vi "convolution.vi"() -> ()   [LabVIEW 2015]
uses:
  <vilib>/vision/NI_Vision_Development_Module.lvlib
panel:
  out "Kernel":dbl[][][](array[numeric])
  out "Image 5":T1(plugin-control)
  out "Image 4":T1(plugin-control)
  out "kernel2":dbl[][](array[numeric])
  out "Divider2":dbl
  out "Divider1":dbl
  out "kernel1":dbl[][](array[numeric])
  out "Image 3":T1(plugin-control)
  out "ImageSize":i32=500
  out "Image":T1(plugin-control)
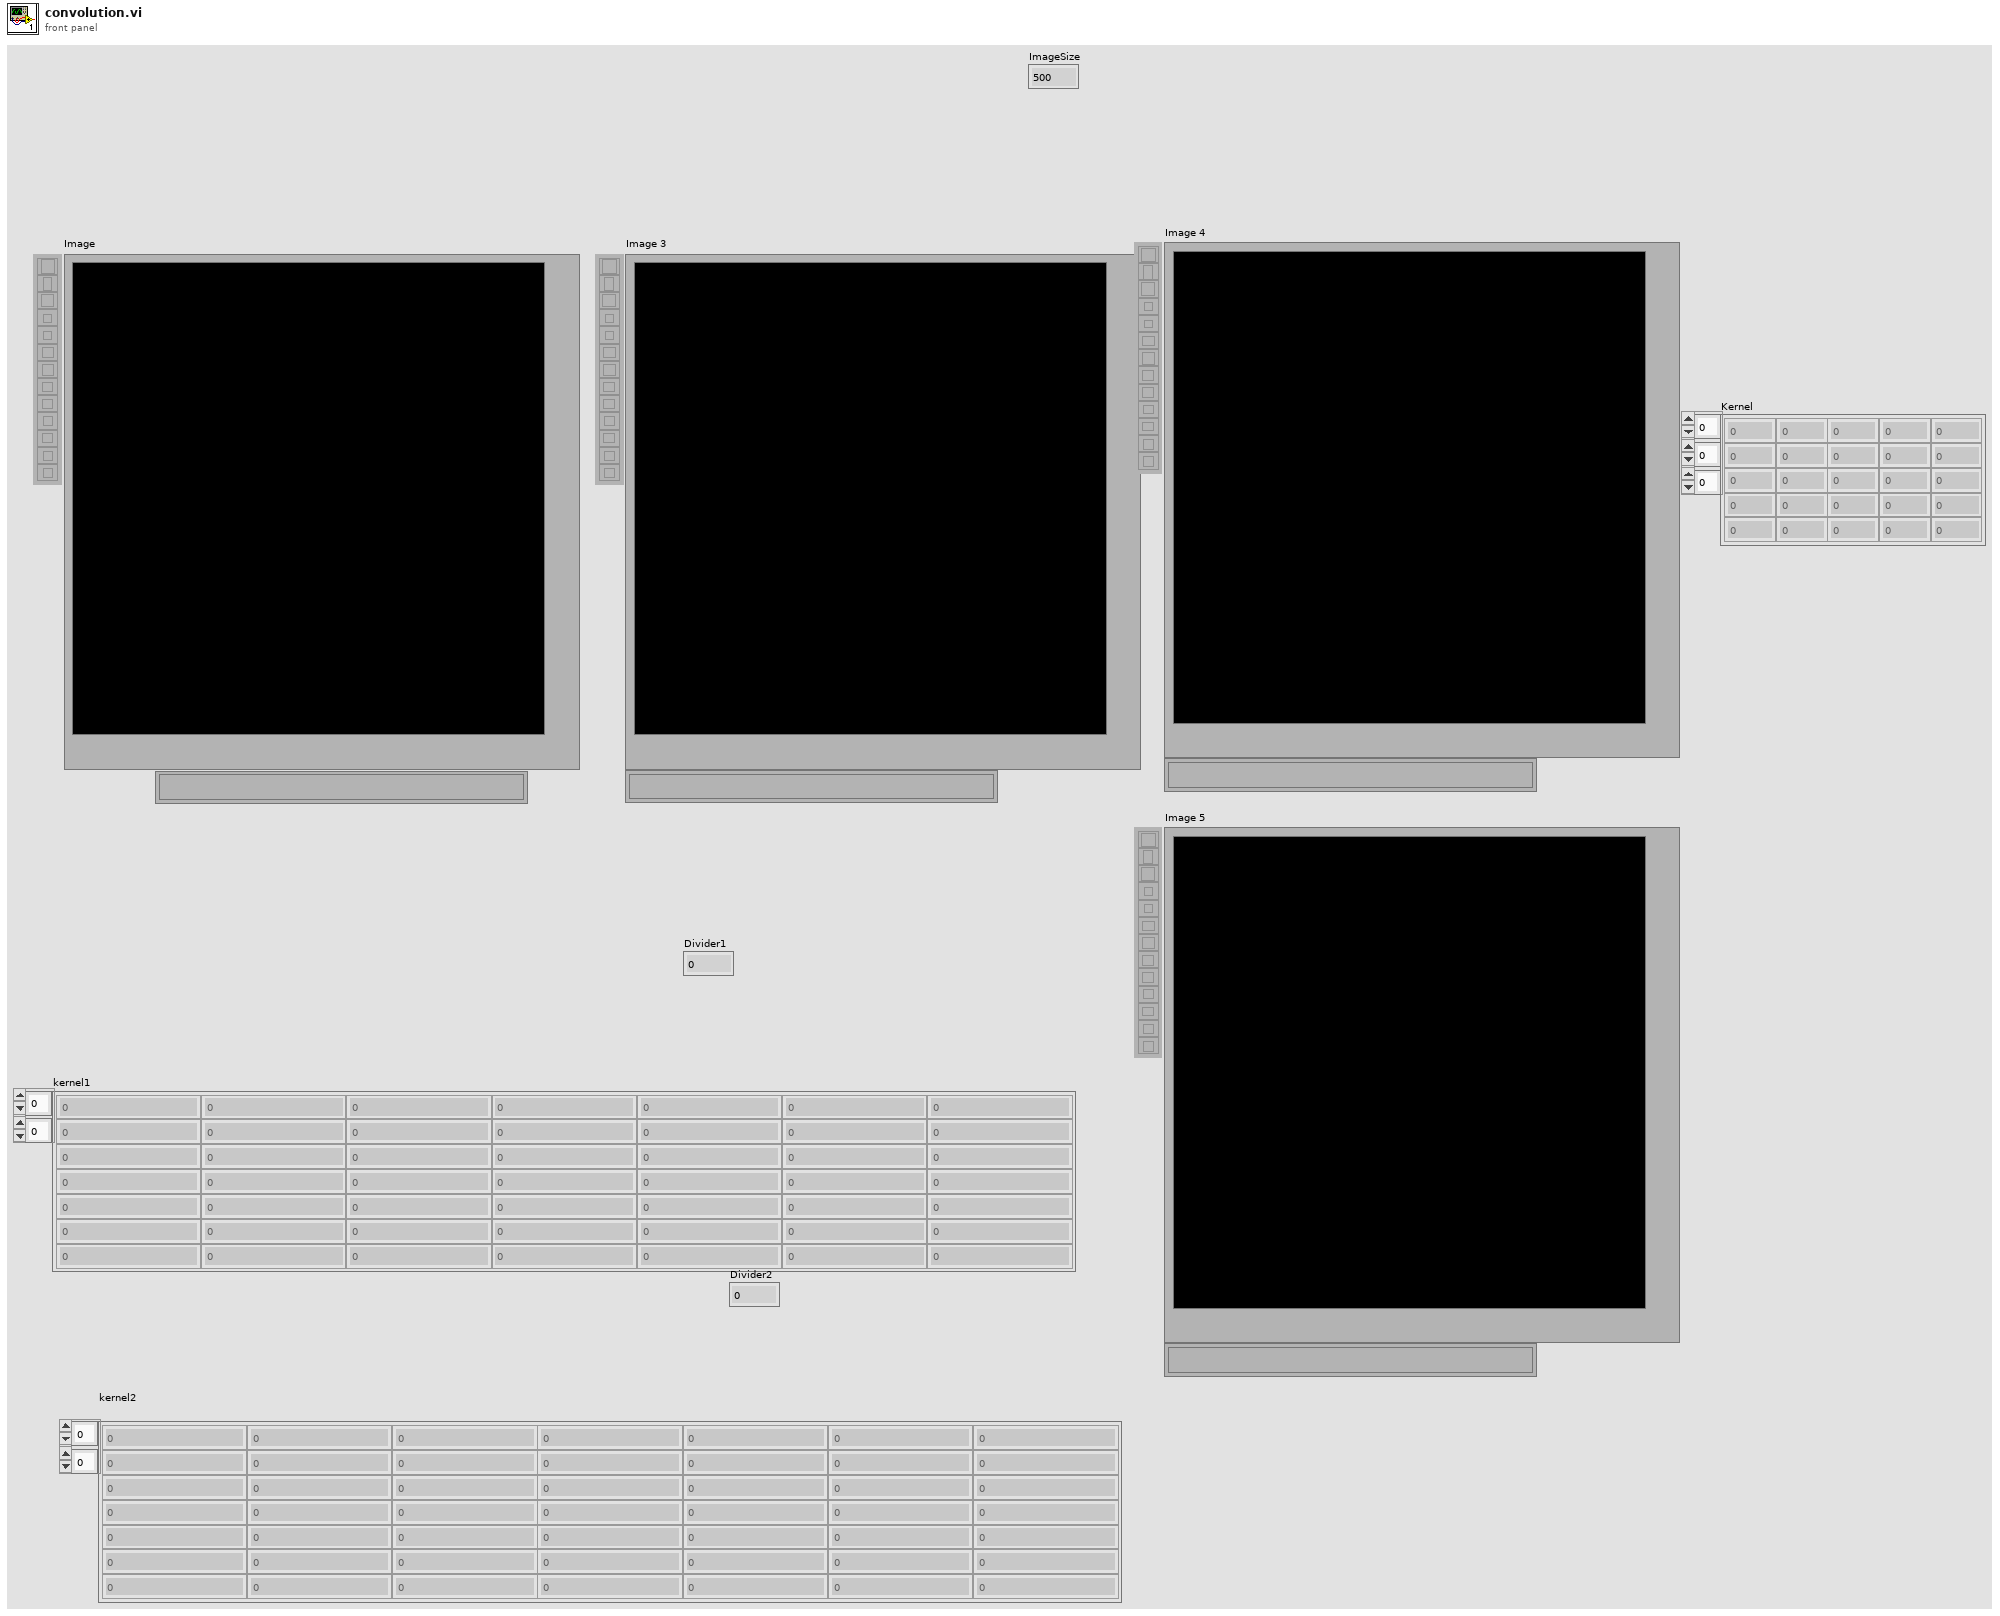
[diagram p1: front panel]
types:
  T1 = typedef "IMAQ Image.ctl" = refnum<image>
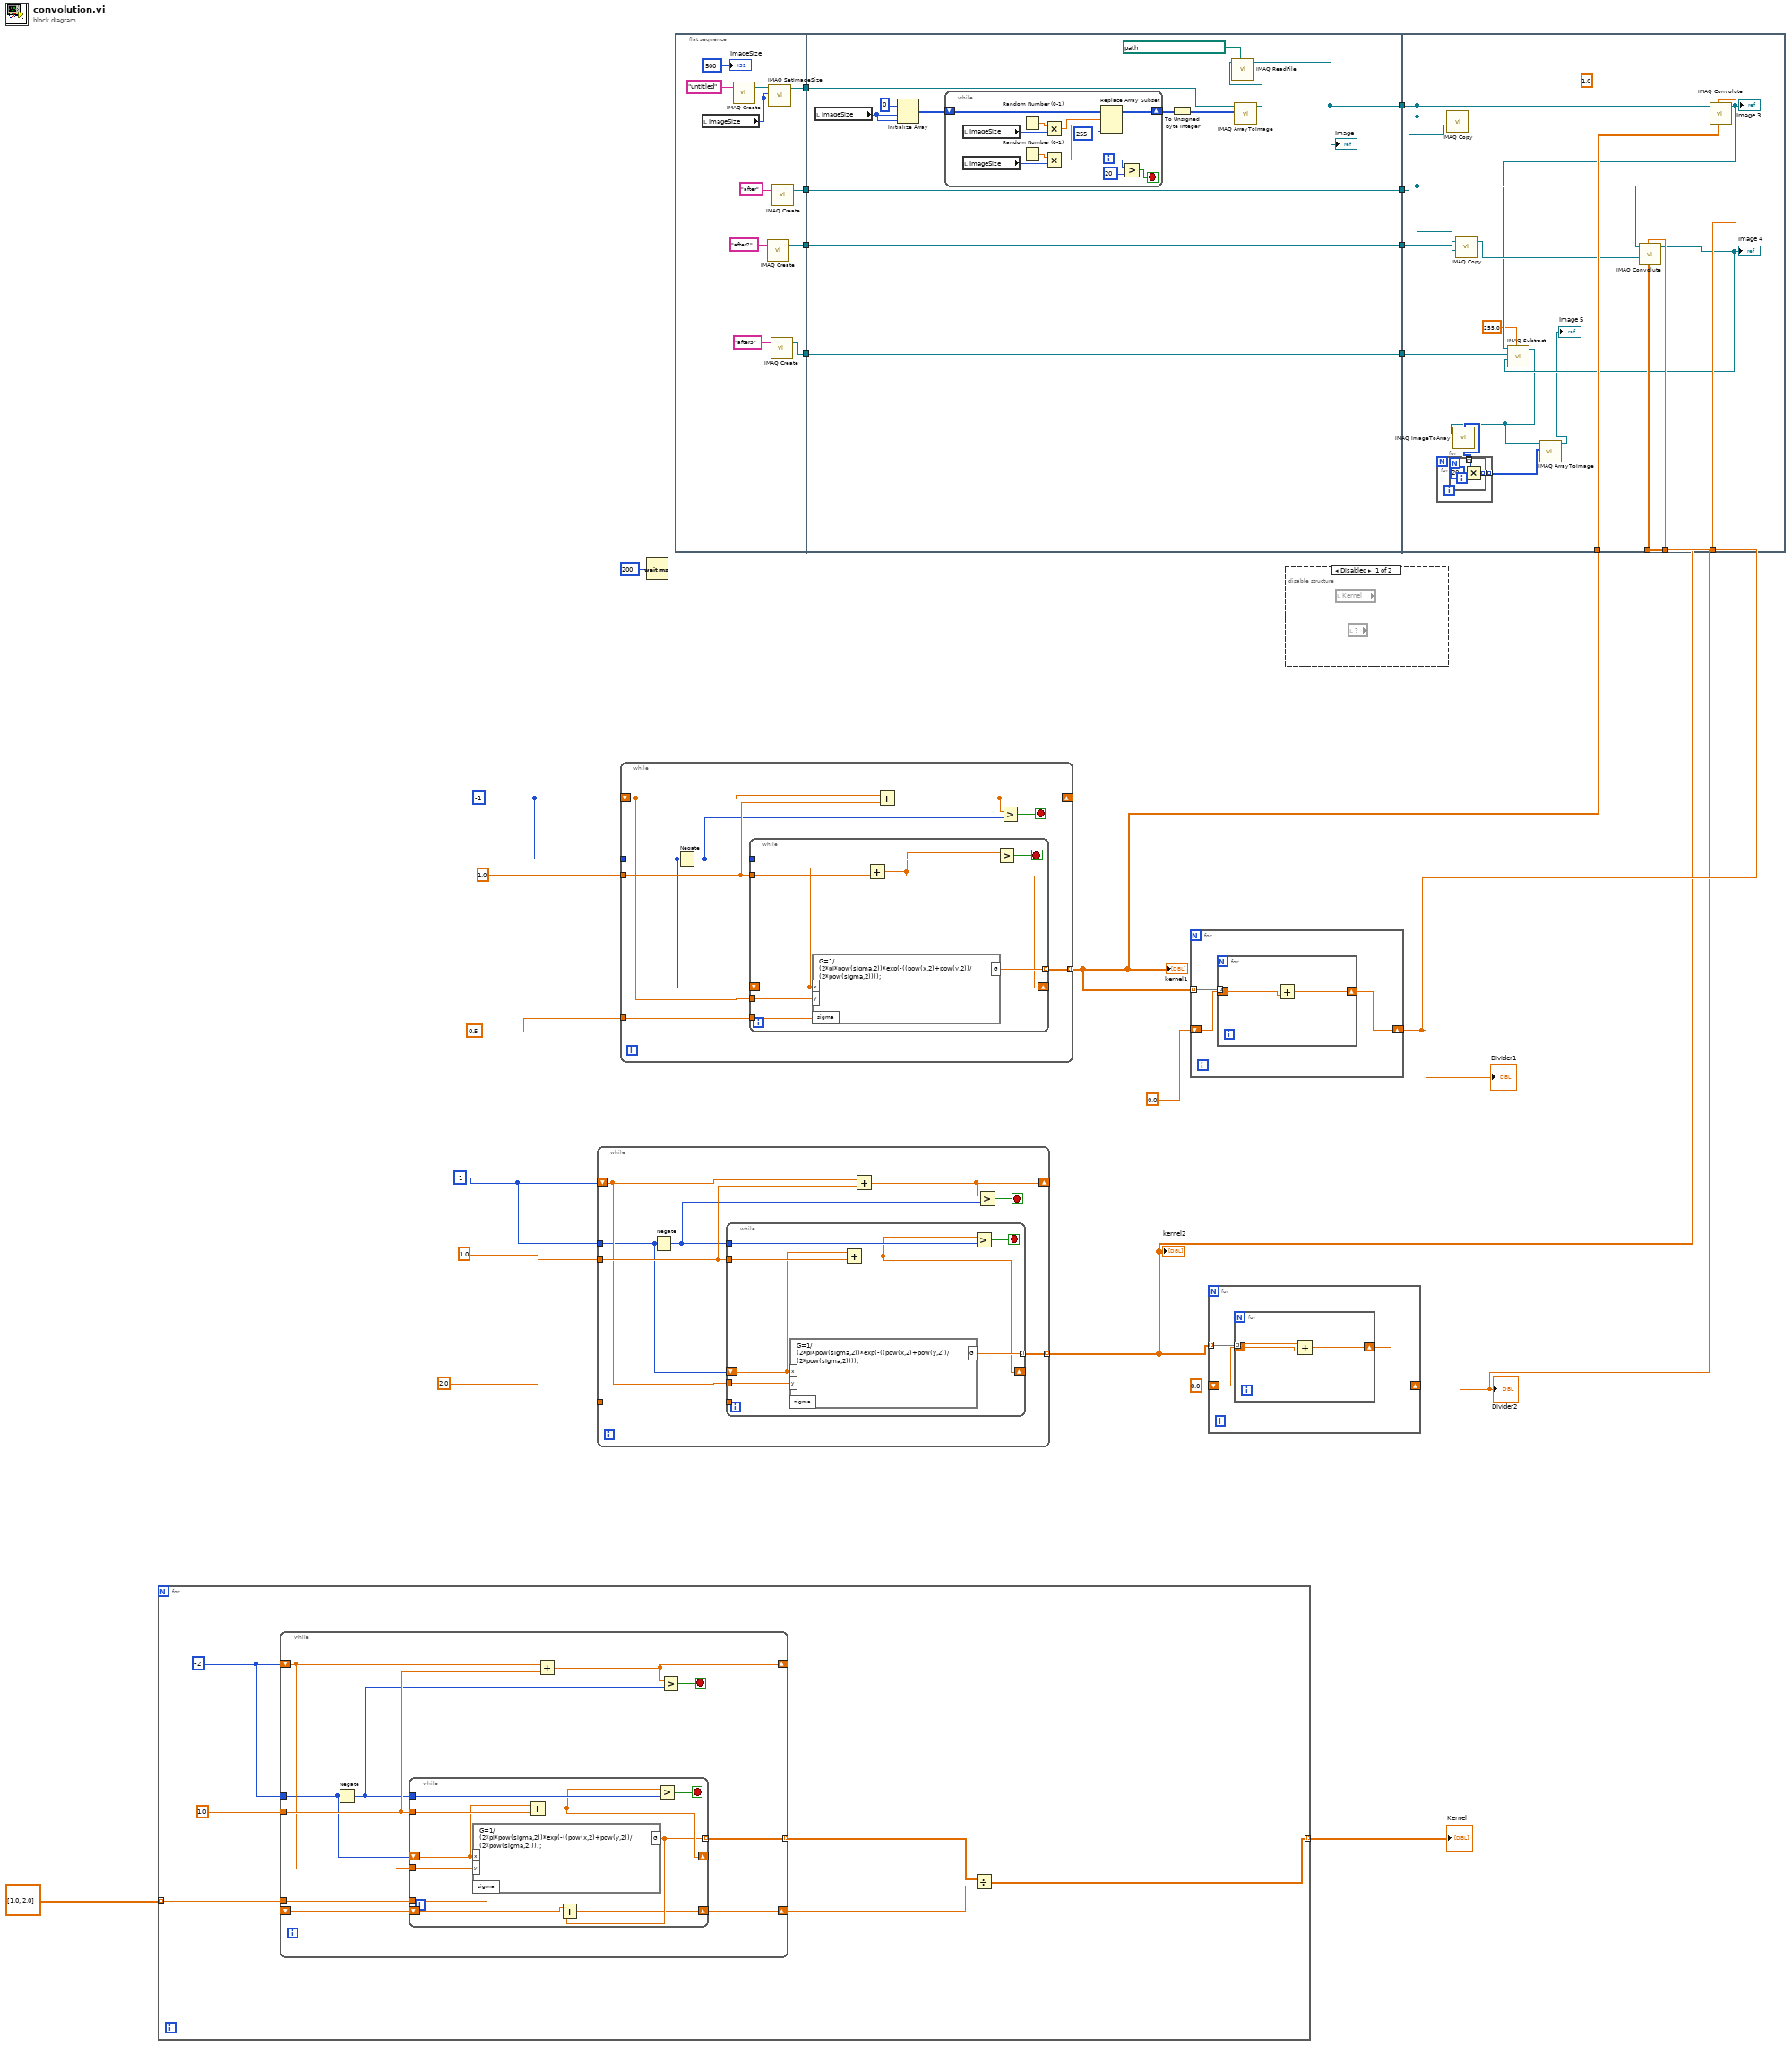
[diagram p0: block diagram]
diagram:
  w10 = -1
  w16 = -1
  n1 = for {
    tunnel: dbl[] [1.0, 2.0] -> [w27] mode=indexing
    tunnel: [w24] -> w1 mode=indexing
    w28 = -2
    n2 = while {
      shift-right: [w34] -> _
      shift-left: w28 -> [w33]
      tunnel: w27 -> [w39]
      tunnel: [w38] -> w26 mode=indexing
      tunnel: 1.0 -> [w37]
      tunnel: w28 -> [w32]
      shift-right: [w30] -> w25
      shift-left: _ -> [w31]
      stop <- w36 stop-if-true
      n3 = Negate(x=w32) -> (-x=w35:i32)
      n4 = while {
        tunnel: w39 -> [w49]
        tunnel: [w41] -> w38 mode=indexing
        tunnel: w37 -> [w48]
        tunnel: w35 -> [w46]
        tunnel: w33 -> [w45]
        shift-right: [w43] -> _
        shift-left: w32 -> [w44]
        shift-right: [w40] -> w30
        shift-left: w31 -> [w42]
        stop <- w47 stop-if-true
        n5 = formula code="G=1/(2*pi*pow(sigma,2))*exp(-((pow(x,2)+pow(y,2))/(2*pow(sigma,2))));"("x"=w44, "sigma"=w49, "y"=w45) -> ("G"=w41:dbl)
        n6 = Add(x=w44, y=w48) -> (x+y=w43:dbl)
        n7 = Add(x=w42, y=w41) -> (x+y=w40:dbl)
        n8 = Greater?(x=w43, y=w46) -> (0:w47:bool)
      }
      n9 = Add(x=w33, y=w37) -> (x+y=w34:dbl)
      n10 = Greater?(x=w34, y=w35) -> (0:w36:bool)
    }
    n11 = Divide(x=w26, y=w25) -> (x/y=w24:dbl[][])
  }
  "Kernel" <- w1
  n12 = while {
    shift-right: [w52] -> _
    shift-left: w10 -> [w51]
    tunnel: 2.0 ("Sigma") -> [w57]
    tunnel: [w56] -> w5 mode=indexing
    tunnel: 1.0 -> [w55]
    tunnel: w10 -> [w50]
    stop <- w54 stop-if-true
    n13 = Negate(x=w50) -> (-x=w53:i32)
    n14 = while {
      tunnel: w57 -> [w65]
      tunnel: [w64] -> w56 mode=indexing
      tunnel: w55 -> [w63]
      tunnel: w53 -> [w61]
      tunnel: w51 -> [w60]
      shift-right: [w58] -> _
      shift-left: w50 -> [w59]
      stop <- w62 stop-if-true
      n15 = formula code="G=1/(2*pi*pow(sigma,2))*exp(-((pow(x,2)+pow(y,2))/(2*pow(sigma,2))));"("x"=w59, "sigma"=w65, "y"=w60) -> ("G"=w64:dbl)
      n16 = Add(x=w59, y=w63) -> (x+y=w58:dbl)
      n17 = Greater?(x=w58, y=w61) -> (0:w62:bool)
    }
    n18 = Add(x=w51, y=w55) -> (x+y=w52:dbl)
    n19 = Greater?(x=w52, y=w53) -> (0:w54:bool)
  }
  "kernel2" <- w5
  n20 = while {
    shift-right: [w68] -> _
    shift-left: w16 -> [w67]
    tunnel: 0.5 ("Sigma") -> [w73]
    tunnel: [w72] -> w15 mode=indexing
    tunnel: 1.0 -> [w71]
    tunnel: w16 -> [w66]
    stop <- w70 stop-if-true
    n21 = Negate(x=w66) -> (-x=w69:i32)
    n22 = while {
      tunnel: w73 -> [w81]
      tunnel: [w80] -> w72 mode=indexing
      tunnel: w71 -> [w79]
      tunnel: w69 -> [w77]
      tunnel: w67 -> [w76]
      shift-right: [w74] -> _
      shift-left: w66 -> [w75]
      stop <- w78 stop-if-true
      n23 = formula code="G=1/(2*pi*pow(sigma,2))*exp(-((pow(x,2)+pow(y,2))/(2*pow(sigma,2))));"("x"=w75, "sigma"=w81, "y"=w76) -> ("G"=w80:dbl)
      n24 = Add(x=w75, y=w79) -> (x+y=w74:dbl)
      n25 = Greater?(x=w74, y=w77) -> (0:w78:bool)
    }
    n26 = Add(x=w67, y=w71) -> (x+y=w68:dbl)
    n27 = Greater?(x=w68, y=w69) -> (0:w70:bool)
  }
  "kernel1" <- w15
  n28 = Wait (ms)(milliseconds to wait=u32 200) -> ()  [unwired: 1 out]
  n29 = flat-sequence {
    tunnel: [w90] -> w22
    tunnel: [w86] -> w21
    tunnel: [w83] -> w7
    tunnel: [w82] -> w4
    tunnel: w22 -> [w99]
    tunnel: w21 -> [w98]
    tunnel: [w95] -> w20
    tunnel: [w98] -> w19
    tunnel: [w94] -> w8
    tunnel: w7 -> [w94]
    tunnel: w4 -> [w93]
    tunnel: [w93] -> w3
    tunnel: w20 -> [w128]
    tunnel: w19 -> [w132]
    tunnel: w15 -> [w131]
    tunnel: w13 -> [w130]
    tunnel: w8 -> [w129]
    tunnel: w6 -> [w126]
    tunnel: w5 -> [w125]
    tunnel: w3 -> [w122]
    frame #0 {
      n30 = local read "ImageSize"() -> (w92:i32)
      n31 = call "IMAQ Create"("Image Name"="untitled") -> ("New Image"=w88:T1)  [unwired: 4 in, 1 out]
      n32 = call "IMAQ Create"("Image Name"="after2") -> ("New Image"=w83:T1)  [unwired: 4 in, 1 out]
      n33 = call "IMAQ SetImageSize"("Y Resolution"=w92, "X Resolution"=w92, "Image"=w88) -> ("Image Out"=w90:T1)  [unwired: 2 in, 1 out]
      n34 = call "IMAQ Create"("Image Name"="after3") -> ("New Image"=w82:T1)  [unwired: 4 in, 1 out]
      n35 = call "IMAQ Create"("Image Name"="after") -> ("New Image"=w86:T1)  [unwired: 4 in, 1 out]
      "ImageSize" <- 500
    }
    frame #1 {
      n36 = local read "ImageSize"() -> (w100:i32)
      n37 = Initialize Array(u8 0 ("element"), w100, w100) -> (w101:u8[][])
      n38 = while {
        shift-right: [w105] -> w104
        shift-left: w101 -> [w109]
        i -> [w116]
        stop <- w114 stop-if-true
        n39 = local read "ImageSize"() -> (w112:i32)
        n40 = local read "ImageSize"() -> (w111:i32)
        n41 = Random Number (0-1)() -> (number: 0 to 1=w113:dbl)
        n42 = Random Number (0-1)() -> (number: 0 to 1=w110:dbl)
        n43 = Multiply(x=w113, y=w112) -> (x*y=w108:dbl)
        n44 = Multiply(x=w110, y=w111) -> (x*y=w107:dbl)
        n45 = Replace Array Subset(array=w109, new element=255 ("new element/subarray"), index (row)=w108, index (col)=w107) -> (w105:u8[][])
        n46 = Greater?(x=w116, y=20) -> (0:w114:bool)
      }
      n47 = To Unsigned Byte Integer(number=w104) -> (unsigned 8bit integer=w103:u8[][])
      n48 = call "IMAQ ArrayToImage"("Image Pixels (U8)"=w103, "Image"=w99) -> ("Image Out"=w96:T1)  [unwired: 8 in, 1 out]
      n49 = call "IMAQ ReadFile"("File Path"=path "E:/[圖片]/IMG_1388.JPG", "Image"=w96) -> ("Image Out"=w95:T1)  [unwired: 5 in, 4 out]
      "Image" <- w95
    }
    frame #2 {
      (unwired) sgl 1.0 ("Divider (kernel sum)")
      n50 = call "IMAQ Copy"("Image Dst"=w132, "Image Src"=w128) -> ("Image Dst Out"=w133:T1)  [unwired: 4 in, 1 out]
      n51 = call "IMAQ Copy"("Image Dst"=w129, "Image Src"=w128) -> ("Image Dst Out"=w127:T1)  [unwired: 4 in, 1 out]
      n52 = call "IMAQ Convolute"("Kernel"=w125, "Divider (kernel sum)"=w126, "Image Dst"=w127, "Image Src"=w128) -> ("Image Dst Out"=w123:T1)  [unwired: 3 in, 4 out]
      "Image 4" <- w123
      n53 = call "IMAQ Convolute"("Kernel"=w131, "Divider (kernel sum)"=w130, "Image Dst"=w133, "Image Src"=w128) -> ("Image Dst Out"=w124:T1)  [unwired: 3 in, 4 out]
      "Image 3" <- w124
      n54 = call "IMAQ Subtract"("Image Src A"=w124, "Constant"=255.0, "Image Dst"=w122, "Image Src B"=w123) -> ("Image Dst Out"=w118:T1)  [unwired: 3 in, 1 out]
      n55 = call "IMAQ ImageToArray"("Image"=w118) -> ("Image Pixels (U8)"=w120:u8[][])  [unwired: 3 in, 4 out]
      n56 = for {
        tunnel: w120 -> [w135] mode=indexing
        tunnel: [w134] -> w119 mode=indexing
        n57 = for {
          tunnel: w135 -> [w138] mode=indexing
          tunnel: [w136] -> w134 mode=indexing
          n58 = Multiply(x=w138, y=u8 20) -> (x*y=w136:u8)
        }
      }
      n59 = call "IMAQ ArrayToImage"("Image Pixels (U8)"=w119, "Image"=w118) -> ("Image Out"=→"Image 5":T1)  [unwired: 8 in, 1 out]
    }
  }
  n60 = for {
    tunnel: w15 -> [w141] mode=indexing
    shift-right: [w139] -> w13
    shift-left: 0.0 -> [w140]
    n61 = for {
      tunnel: w141 -> [w144] mode=indexing
      shift-right: [w142] -> w139
      shift-left: w140 -> [w143]
      n62 = Add(x=w144, y=w143) -> (x+y=w142:dbl)
    }
  }
  "Divider1" <- w13
  n63 = for {
    tunnel: w5 -> [w147] mode=indexing
    shift-right: [w145] -> w6
    shift-left: 0.0 -> [w146]
    n64 = for {
      tunnel: w147 -> [w150] mode=indexing
      shift-right: [w148] -> w145
      shift-left: w146 -> [w149]
      n65 = Add(x=w150, y=w149) -> (x+y=w148:dbl)
    }
  }
  "Divider2" <- w6
  n66 = disable-structure shown="Disabled" {
    frame Disabled {
      n67 = local read "Kernel"() -> ()  [unwired: 1 out]
      n68 = local read item#-1() -> ()  [unwired: 1 out]
    }
    frame Enabled {
    }
  }
